vi "CheckThorlabsAB.vi"() -> ()   [LabVIEW 2019, in "Instrument.Temperhum.lvclass"]
uses:
  Instrument.Temperhum.lvclass
  Temperhum.Thorlabs/Temperhum.Thorlabs.lvclass
  C:/Users/Ranjani/Documents/GitHub/Temperhum-Instrument/lvsrc/SMOs/Instrument.Temperhum/Instrument.Temperhum.lvclass
  Temperhum.PCSensor/Temperhum.PCSensor.lvclass
panel:
  in  "Enum":enum16{"parent", "thorlabs", "pc sensor"}(ring)
  out "error out":errorcluster
  in  "error in (no error)":errorcluster
  out "Humidity (%RH)":dbl
  out "Temperature (K)":dbl
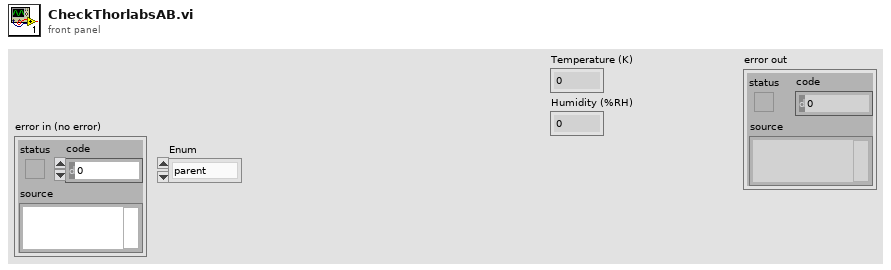
[diagram p1: front panel]
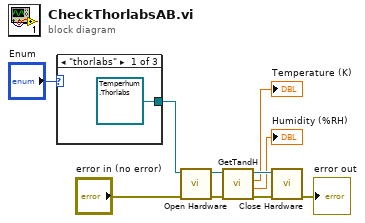
[diagram p0: block diagram]
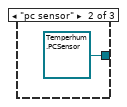
[diagram p2: hidden frame]
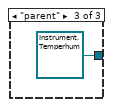
[diagram p3: hidden frame]
diagram:
  n1 = case shown="\"thorlabs\"" "Enum" {
    tunnel: [refnum<class "Temperhum.Thorlabs.lvclass"> refnum ("Temperhum.Thorlabs.lvclass") refnum<class "Temperhum.PCSensor.lvclass"> refnum ("Temperhum.PCSensor.lvclass") refnum<class "Instrument.Temperhum.lvclass"> refnum ("Instrument.Temperhum.lvclass")] -> w1
    frame "thorlabs" {
    }
    frame "pc sensor" {
    }
    frame "parent" {
    }
  }
  n2 = call-dynamic "Open Hardware.vi"("error in (no error)"="error in (no error)", "Instrument.FrameworkTemplate"=w1) -> ("error out"=w5:errorcluster, "Instrument.FrameworkTemplate out"=w10:refnum<class "Instrument.Temperhum.lvclass">)  [unwired: 8 in]
  n3 = call-dynamic "GetTandH.vi"("error in (no error)"=w5, "Instrument.Temperhum in"=w10) -> ("error out"=w4:errorcluster, "Humidity (%RH)"=→"Humidity (%RH)":dbl, "Temperature (K)"=→"Temperature (K)":dbl, "Instrument.Temperhum out"=w9:refnum<class "Instrument.Temperhum.lvclass">)  [unwired: 6 in]
  n4 = call-dynamic "Close Hardware.vi"("error in (no error)"=w4, "Instrument.FrameworkTemplate"=w9) -> ("error out"=→"error out":errorcluster)  [unwired: 8 in, 1 out]
